vi "sv_Convert to Even Angle Signal (Generic) with IC.vi"(0 "scaled signal [EU]":dbl[](array[numeric]), 2 "reset? (F)":bool, 5 "sampling rate [Hz]":dbl=1.0, 7 "speed position info":T3, 9 "channel count":i32, 11 "initial conditions":T1={"filter prototype"={"left wing"=[], "increment"=[], "max dec"=128, "timing jitter"=enum."Interpolation", "band limiting?"=TRUE}, "interpolation filter state"={"corrected lengths"=[], "initH"=[]}, "resample state"={"signal length"=0, "time"=[], "reset state"=FALSE, "state"={"init condition"=[], "start index"=0, "channel count"=0, "condition len"=0, "position"=0.0, "time interval"=0.0, "max cond len"=0}, "offset"=0.0}} {"filter prototype"."increment" format="%.2f"; "filter prototype"."left wing" format="%.2f"}, 12 "max order":dbl=16.0) -> (4 "generic even-angle signal":dbl[][](array[numeric]), 6 "generic position info":dbl[](array[numeric]), 8 "offset":dbl, 10 "pulse/revolution":dbl, 15 "final conditions":T1={"filter prototype"={"left wing"=[], "increment"=[], "max dec"=128, "timing jitter"=enum."Interpolation", "band limiting?"=TRUE}, "interpolation filter state"={"corrected lengths"=[], "initH"=[]}, "resample state"={"signal length"=0, "time"=[], "reset state"=FALSE, "state"={"init condition"=[], "start index"=0, "channel count"=0, "condition len"=0, "position"=0.0, "time interval"=0.0, "max cond len"=0}, "offset"=0.0}} {"filter prototype"."increment" format="%.2f"; "filter prototype"."left wing" format="%.2f"})   [LabVIEW 2017, in "SoundVib_Resampling.lvlib"]
doc: "Converts an even-time-spaced scaled signal to an even-angle-spaced signal by resampling the acquired signal. The output signal is synchronous to the rotational speed with a constant number of samples per revolution. Use this VI on embedded targets that have limited computational resources. Wire data to the <B>scaled signal [EU]</B> input to determine the polymorphic instance to use or manually select the instance."
uses:
  <vilib>/addons/Sound and Vibration/Order Analysis/Resample Order Tracking/SoundVib_Resampling.lvlib
  <vilib>/addons/Sound and Vibration/Order Analysis/Misc/OAT Position Info.ctl
  <vilib>/addons/_NISVFA/_Shared subVIs/Controls/svc_Convert to Even Angle State.ctl
  <vilib>/addons/_NISVFA/_Shared subVIs/Controls/OAT Resample Filter Prototype.ctl
  <vilib>/addons/Sound and Vibration/Order Analysis/Adv Resampling/oa_Adjust Resample State Info.vi
  <vilib>/addons/Sound and Vibration/Order Analysis/Adv Resampling/OAT LP Kaiser Window Design.vi
  <vilib>/addons/Sound and Vibration/Order Analysis/Resample Order Tracking/SubVIs/oa_CIC Filter Length.vi
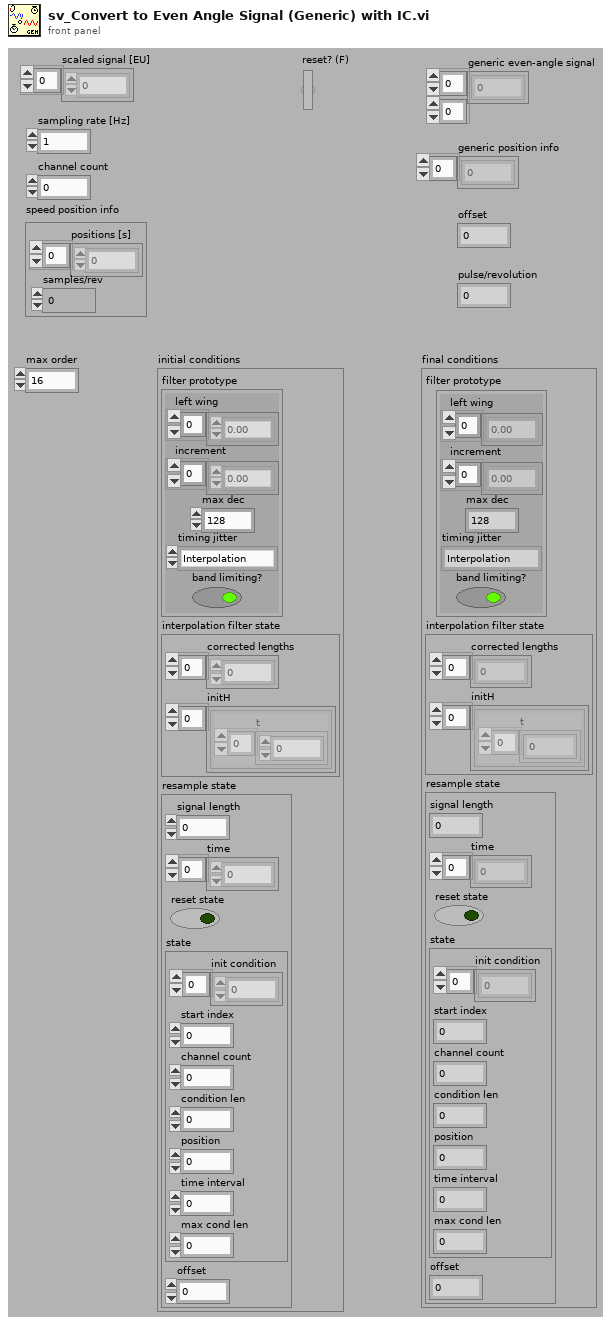
[diagram p1: front panel]
types:
  T1 = typedef "svc_Convert to Even Angle State.ctl" = cluster{"filter prototype":T2, "interpolation filter state":cluster{"corrected lengths":i32[], "initH":cluster{"t":dbl[]}[]}, "resample state":cluster{"signal length":u64, "time":dbl[], "reset state":bool, "state":cluster{"init condition":dbl[], "start index":i32, "channel count":i32, "condition len":i32, "position":dbl, "time interval":dbl, "max cond len":i32}, "offset":dbl}}
  T2 = typedef "OAT Resample Filter Prototype.ctl" = cluster{"left wing":dbl[], "increment":dbl[], "max dec":i32, "timing jitter":enum32{"Interpolation", "Rounding"}, "band limiting?":bool}
  T3 = typedef "OAT Position Info.ctl" = cluster{"positions [s]":dbl[], "samples/rev":dbl}
  T4 = cluster{"interpolation/decimation factor":i32, "stages":i32, "lag":i32}
  T5 = cluster{"corrected lengths":i32[], "initH":cluster{"t":dbl[]}[]}
  T6 = cluster{"signal length":u64, "time":dbl[], "reset state":bool, "state":cluster{"init condition":dbl[], "start index":i32, "channel count":i32, "condition len":i32, "position":dbl, "time interval":dbl, "max cond len":i32}, "offset":dbl}
  T7 = cluster{"interpolation/decimation factor":i32, "stages":i32, "lag":i32}[]
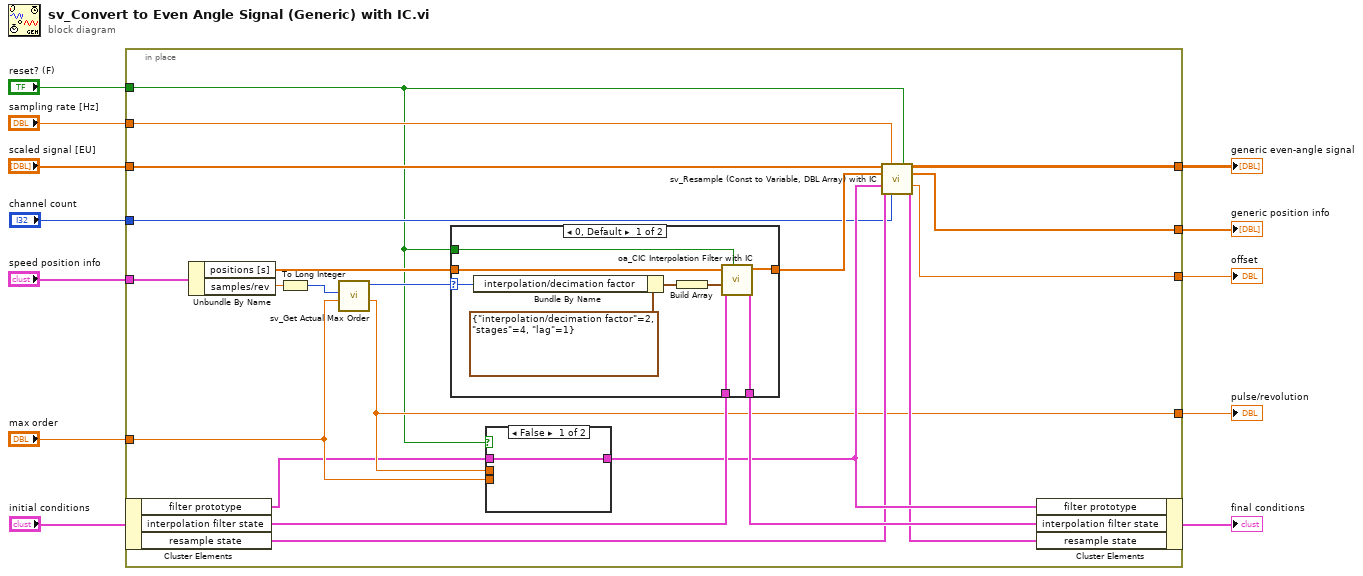
[diagram p0: block diagram]
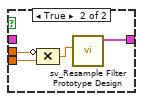
[diagram p2: hidden frame]
diagram:
  n1 = in-place {
    in-place-border: "max order" -> [w33]
    in-place-border: "speed position info" -> [w32]
    in-place-border: "sampling rate [Hz]" -> [w29]
    in-place-border: "scaled signal [EU]" -> [w28]
    in-place-border: "reset? (F)" -> [w14]
    in-place-border: [w19] -> w5
    in-place-border: [w18] -> w4
    in-place-border: [w17] -> w3
    in-place-border: [w16] -> w2
    in-place-border: "channel count" -> [w15]
    n2 = in-place-cluster #1("initial conditions") -> ("filter prototype"=w13:T2, "interpolation filter state"=w24:T5, "resample state"=w21:T6)
    n3 = Unbundle By Name(w32) -> ("positions [s]"=w27:dbl[], "samples/rev"=w31:dbl)
    n4 = To Long Integer(number=w31) -> (32bit integer=w30:i32)
    n5 = call <vilib>:"sv_Get Actual Max Order.vi"("max order"=w33, "pulse/revolution (1)"=w30) -> ("new pulse/revolution"=w17:dbl, "interpolation factor"=w25:i32)  [unwired: 8 in]
    n6 = case shown="0, Default" w25 {
      selector: w25 -> [w41 _]
      tunnel: w27 -> [w47 w49]
      tunnel: [w46 w49] -> w26
      tunnel: w14 -> [w45 _]
      tunnel: w24 -> [w40 w48]
      tunnel: [w39 w48] -> w23
      frame 0, Default {
        n7 = Bundle By Name(cluster=T4 {"interpolation/decimation factor"=2, "stages"=4, "lag"=1} ("CIC filter settings"), "interpolation/decimation factor"=w41) -> (w43:T4)
        n8 = Build Array(w43) -> (w42:T7)
        n9 = call <vilib>:"oa_CIC Interpolation Filter with IC.vi"("reset? (True)"=w45, "initial conditions"=w40, "CIC filter settings"=w42, "X"=w47) -> ("final conditions"=w39:T5, "Y"=w46:dbl[])  [unwired: 5 in, 1 out]
      }
      frame 1 {
      }
    }
    n10 = case shown="False" w14 {
      tunnel: w33 -> [_ w38]
      tunnel: [w34 w36] -> w22
      tunnel: w17 -> [_ w35]
      tunnel: w13 -> [w34 _]
      frame False {
      }
      frame True {
        n11 = Compound Arithmetic op=MULTIPLY(invert w35, w38) -> (w37:dbl)
        n12 = call <vilib>:"sv_Resample Filter Prototype Design.vi"("rolloff"=w37) -> ("filter prototype out"=w36:T2)  [unwired: 10 in]
      }
    }
    n13 = call <vilib>:"sv_Resample (Const to Variable, DBL Array) with IC.vi"("Array"=w28, "sampling rate"=w29, "reset? (True)"=w14, "time"=w26, "filter prototype"=w22, "initial conditions"=w21, "channel count"=w15) -> ("Y"=w19:dbl[][], "time stamps"=w18:dbl[], "offset"=w16:dbl, "final conditions"=w20:T6)  [unwired: 5 in]
    n14 = in-place-cluster #1("filter prototype"=w22, "interpolation filter state"=w23, "resample state"=w20) -> (→"final conditions":T1)
  }
  "generic even-angle signal" <- w5
  "generic position info" <- w4
  "pulse/revolution" <- w3
  "offset" <- w2
